vi "Ref plots core.vi"(0 "Snapshot file path":path, 1 "Snapshot":bool, 2 "Initialise":bool, 5 "Ref Test Data in in":dbl[][](array[numeric]), 9 "Reset Graphs":bool, 11 "error in (no error)":errorcluster, 12 "Buffer Size":i32, 13 "Refresh rate (ms)":u32=200 min=10 step=10) -> (4 "Ref Test Data out":dbl[][](array[numeric]), 6 "Actual refresh rate (ms)":u32, 10 "Graphs cluster":T1, 15 "error":errorcluster)   [LabVIEW 2017]
uses:
  Typedefs/Ref plot graphs cluster.ctl
panel:
  out "Refresh rate (ms)":u32=200 min=10 step=10
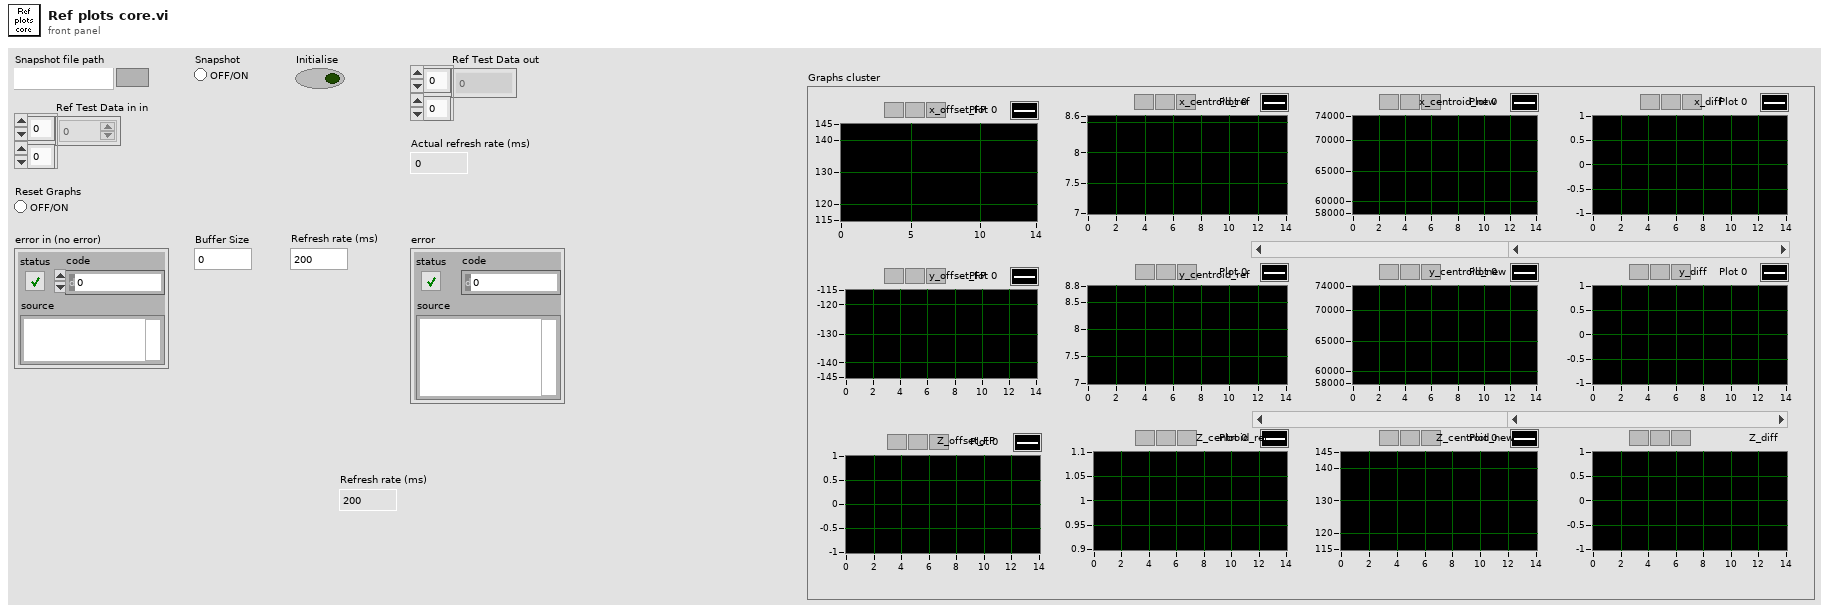
[diagram p1: front panel]
types:
  T1 = typedef "Ref plot graphs cluster.ctl" = cluster{"x_offset_FP":dbl[], "y_offset_FP":dbl[], "x_centroid_ref":dbl[], "y_centroid_ref":dbl[], "x_centroid_new":dbl[], "y_centroid_new":dbl[], "x_diff":dbl[], "y_diff":dbl[], "Z_offset_FP":dbl[], "Z_centroid_ref":dbl[], "Z_centroid_new":dbl[], "Z_diff":dbl[]}
  T2 = enum32{"Invalid", "Standard", "Closed", "Hidden", "Minimized", "Maximized"}
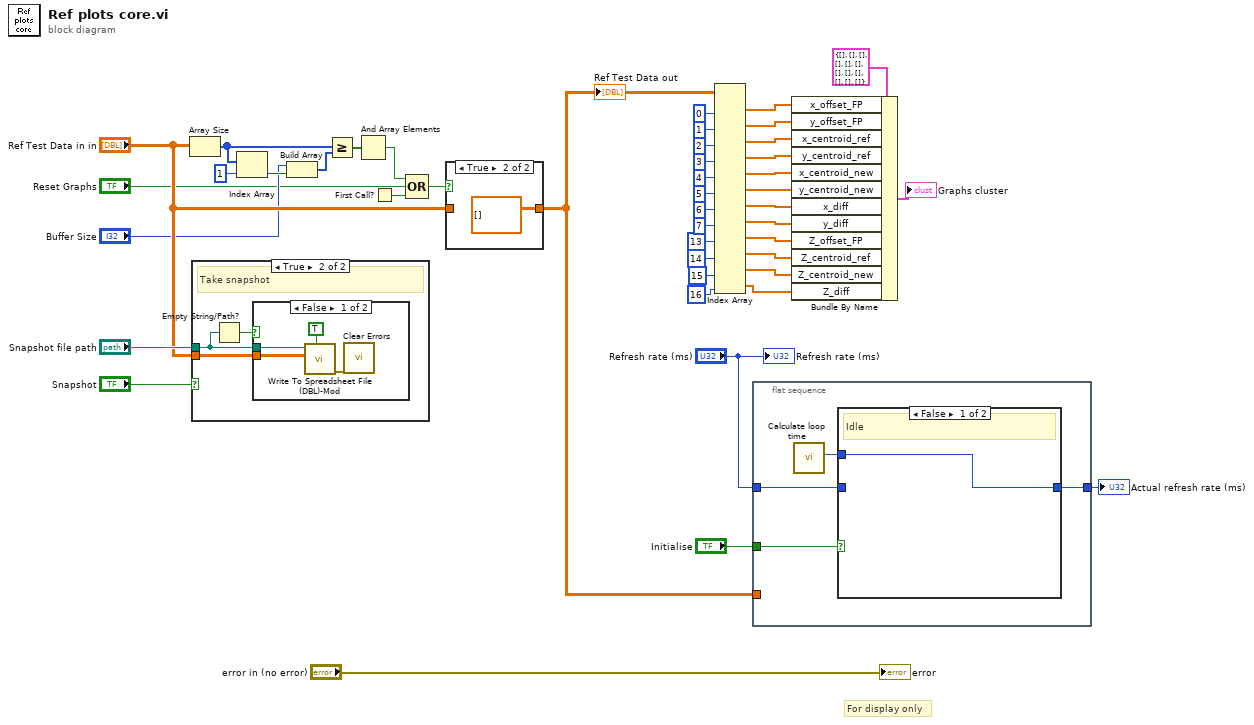
[diagram p0: block diagram]
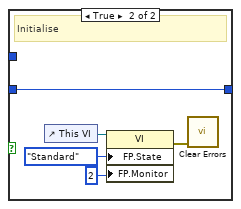
[diagram p2: hidden frame]
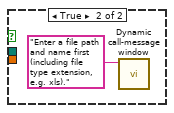
[diagram p5: hidden frame]
diagram:
  # "For display only"
  n1 = Array Size(array="Ref Test Data in in") -> (size(s)=w42:i32[])
  n2 = case shown="True" "Snapshot" {
    tunnel: "Ref Test Data in in" -> [_ w47]
    tunnel: "Snapshot file path" -> [_ w46]
    frame False {
      # "Idle"
    }
    frame True {
      # "Take snapshot"
      n3 = Empty String/Path?(string/path=w46) -> (empty?=w45:bool)
      n4 = case shown="False" w45 {
        tunnel: w47 -> [w51 _]
        tunnel: w46 -> [w48 _]
        frame False {
          n5 = call <userlib>:"Write To Spreadsheet File (DBL)-Mod.vi"("append to file? (new file:F)"=TRUE, "2D data"=w51, "file path (dialog if empty)"=w48) -> ("error out"=w50:errorcluster)  [unwired: 7 in, 1 out]
          n6 = call <vilib>:"Clear Errors.vi"("error in (no error)"=w50) -> ()  [unwired: 5 in, 2 out]
        }
        frame True {
          n7 = call "Dynamic call-message window.vi"("Message"="Enter a file path and name first (including file type extension, e.g. xls).") -> ()  [unwired: 10 in, 1 out]
        }
      }
    }
  }
  n8 = Index Array(array=w42, index=1) -> (element=w44:i32)
  n9 = Build Array("Buffer Size", w44) -> (w39:i32[])
  n10 = Greater Or Equal?(x=w42, y=w39) -> (x >= y?=w40:bool[])
  n11 = And Array Elements(Boolean array=w40) -> (logical AND=w41:bool)
  n12 = First Call?() -> (First Call?: T/F=w38:bool)
  n13 = Compound Arithmetic op=OR(w41, "Reset Graphs", w38) -> (w37:bool)
  n14 = case shown="True" w37 {
    tunnel: "Ref Test Data in in" -> [w53 _]
    tunnel: [w53 dbl[][] []] -> w3
    frame False {
    }
    frame True {
    }
  }
  "Ref Test Data out" <- w3
  n15 = Index Array(array=w3, index (col) #1=0 ("disabled index (col)"), index (col) #2=1 ("index (col)"), index (col) #3=2 ("index (col)"), index (col) #4=3 ("index (col)"), index (col) #5=4 ("index (col)"), index (col) #6=5 ("index (col)"), index (col) #7=6 ("index (col)"), index (col) #8=7 ("index (col)"), index (col) #9=13 ("index (col)"), index (col) #10=14 ("index (col)"), index (col) #11=15 ("index (col)"), index (col) #12=16 ("index (col)")) -> (element #1=w16:dbl[], element #2=w15:dbl[], element #3=w14:dbl[], element #4=w13:dbl[], element #5=w12:dbl[], element #6=w11:dbl[], element #7=w10:dbl[], element #8=w9:dbl[], element #9=w8:dbl[], element #10=w7:dbl[], element #11=w6:dbl[], element #12=w1:dbl[])  [unwired: 12 in]
  n16 = flat-sequence {
    tunnel: "Initialise" -> [w58]
    tunnel: [w57] -> w30
    tunnel: "Refresh rate (ms)" -> [w56]
    tunnel: w3 -> [_]
    frame #0 {
      n17 = call <userlib>:"Calculate loop time.vi"() -> ("Loop time (ms)"=w55:u32)  [unwired: 11 in]
      n18 = case shown="False" w58 {
        tunnel: [w59 w60] -> w57
        tunnel: w56 -> [_ w60]
        tunnel: w55 -> [w59 _]
        frame False {
          # "Idle"
        }
        frame True {
          # "Initialise"
          n19 = control-ref of="This VI"() -> (w64:refnum<vi>)
          n20 = property class="VI"(reference=w64, "FP.State"=T2."Standard" ("Front Panel Window:State"), "FP.Monitor"=u16 2 ("Front Panel Window:Monitor")) -> (error out=w61:errorcluster)  [unwired: 1 in, 1 out]
          n21 = call <vilib>:"Clear Errors.vi"("error in (no error)"=w61) -> ()  [unwired: 5 in, 2 out]
        }
      }
    }
  }
  n22 = Bundle By Name(cluster=T1 {"x_offset_FP"=[], "y_offset_FP"=[], "x_centroid_ref"=[], "y_centroid_ref"=[], "x_centroid_new"=[], "y_centroid_new"=[], "x_diff"=[], "y_diff"=[], "Z_offset_FP"=[], "Z_centroid_ref"=[], "Z_centroid_new"=[], "Z_diff"=[]} ("Graphs cluster"), "x_offset_FP"=w16, "y_offset_FP"=w15, "x_centroid_ref"=w14, "y_centroid_ref"=w13, "x_centroid_new"=w12, "y_centroid_new"=w11, "x_diff"=w10, "y_diff"=w9, "Z_offset_FP"=w8, "Z_centroid_ref"=w7, "Z_centroid_new"=w6, "Z_diff"=w1) -> (→"Graphs cluster":T1)
  "Refresh rate (ms)" <- "Refresh rate (ms)"
  "Actual refresh rate (ms)" <- w30
  "error" <- "error in (no error)"
